vi "SCA_Query.vi"(0 "System no.":i32=1 min=1 max=4 step=1, 5 "error in":errorcluster) -> (14 "Axis 1":string, 15 "Axis 2":string, 19 "error out":errorcluster)   [LabVIEW 2020]
doc: "Indicates which axes can be controlled with controller keyboard cursor keys: left-right for axis 1 and up-down for axis 2."
uses:
  Global1.vi
panel:
  # "Indicates which axes can be controlled with the controller\nkeyboard keys, left right for axis 1 and up down for axis 2."
  # "Cursor controlled"
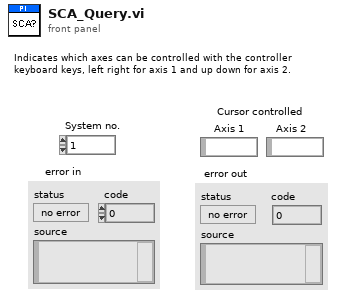
[diagram p1: front panel]
types:
  T1 = typedef "Syntax.ctl" = enum16{"GCS 1.0", "GCS 2.0", "GCS 3.0"}
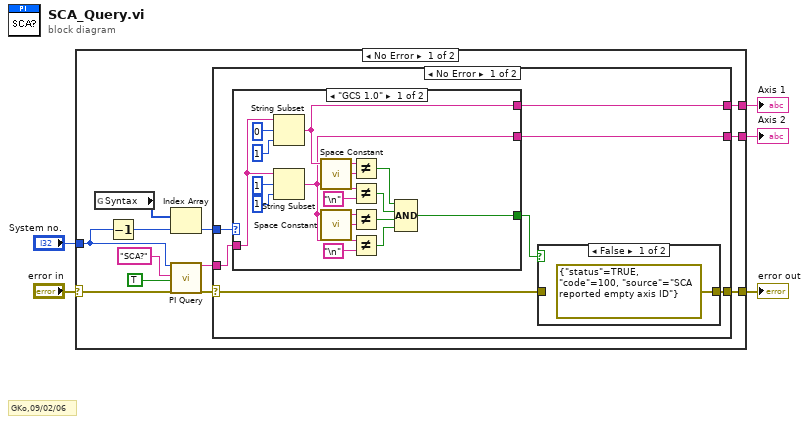
[diagram p0: block diagram]
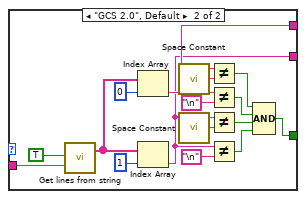
[diagram p2: hidden frame]
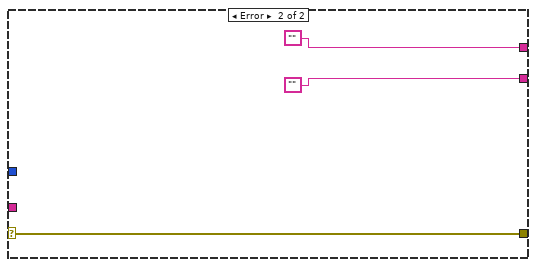
[diagram p4: hidden frame]
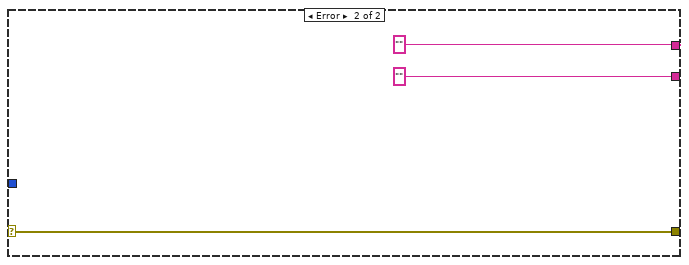
[diagram p5: hidden frame]
diagram:
  # "GKo,09/02/06"
  n1 = case shown="No Error" "error in" {
    selector: "error in" -> [w7 w62]
    tunnel: "System no." -> [w11 _]
    tunnel: [w16 ""] -> w4
    tunnel: [w15 ""] -> w3
    tunnel: [w14 w62] -> w2
    frame No Error {
      n2 = global read "Global1.vi" "Syntax"() -> (w12:T1[])
      n3 = Decrement(x=w11) -> (x-1=w13:i32)
      n4 = Index Array(array=w12, index=w13) -> (element=w10:T1)
      n5 = call "PI Query.vi"("System no."=w11, "String to send"="SCA?", "Attach termination char.?"=TRUE ("Attach Linefeed?"), "error in"=w7) -> ("String read"=w9:string, "error out"=w8:errorcluster)  [unwired: 3 in, 11 out]
      n6 = case shown="No Error" w8 {
        selector: w8 -> [w18 w59]
        tunnel: w9 -> [w24 _]
        tunnel: [w22 ""] -> w16
        tunnel: [w21 ""] -> w15
        tunnel: [w20 w59] -> w14
        tunnel: w10 -> [w19 _]
        frame No Error {
          n7 = case shown="\"GCS 1.0\"" w19 {
            tunnel: w24 -> [w32 w46]
            tunnel: [w27 w48] -> w23
            tunnel: [w26 w44] -> w22
            tunnel: [w25 w41] -> w21
            frame "GCS 1.0" {
              n8 = String Subset(string=w32, offset (0)=0, length (rest)=1 ("length")) -> (substring=w26:string)
              n9 = String Subset(string=w32, offset (0)=1, length (rest)=1 ("length")) -> (substring=w25:string)
              n10 = call "Space Constant.vi"() -> ("String"=w39:string)
              n11 = call "Space Constant.vi"() -> ("String"=w35:string)
              n12 = Not Equal?(x=w26, y=w39) -> (x != y?=w31:bool)
              n13 = Not Equal?(x=w26, y="\n") -> (x != y?=w30:bool)
              n14 = Not Equal?(x=w25, y=w35) -> (x != y?=w29:bool)
              n15 = Not Equal?(x=w25, y="\n") -> (x != y?=w28:bool)
              n16 = Compound Arithmetic op=AND(w31, w30, w29, w28) -> (w27:bool)
            }
            frame "GCS 2.0", Default {
              n17 = call "Get lines from string.vi"("Cut spaces?"=TRUE, "Input string"=w46) -> ("Strings"=w43:string[])  [unwired: 1 in, 16 out]
              n18 = Index Array(array=w43, index=0) -> (element=w44:string)
              n19 = Index Array(array=w43, index=1) -> (element=w41:string)
              n20 = call "Space Constant.vi"() -> ("String"=w56:string)
              n21 = call "Space Constant.vi"() -> ("String"=w54:string)
              n22 = Not Equal?(x=w44, y=w56) -> (x != y?=w52:bool)
              n23 = Not Equal?(x=w44, y="\n") -> (x != y?=w51:bool)
              n24 = Not Equal?(x=w41, y=w54) -> (x != y?=w50:bool)
              n25 = Not Equal?(x=w41, y="\n") -> (x != y?=w49:bool)
              n26 = Compound Arithmetic op=AND(w52, w51, w50, w49) -> (w48:bool)
            }
          }
          n27 = case shown="False" w23 {
            tunnel: [errorcluster {"status"=TRUE, "code"=100, "source"="SCA reported empty axis ID"} ("error out") w58] -> w20
            tunnel: w18 -> [_ w58]
            frame False {
            }
            frame True {
            }
          }
        }
        frame Error {
        }
      }
    }
    frame Error {
    }
  }
  "error out" <- w2
  "Axis 1" <- w4
  "Axis 2" <- w3
